vi "Function_Clamp #.vi"(8 "Error in":errorcluster, 9 "CoordSys In":T3 {"Measurement System"."Axis Reference" items=["Direct", "Indirect"]; "Measurement System"."Angle (deg)" format="%.2f"; "Measurement System"."Origin"."Y" format="%.2f"; "Measurement System"."Origin"."X" format="%.2f"; "Reference System"."Axis Reference" items=["Direct", "Indirect"]; "Reference System"."Angle (deg)" format="%.2f"; "Reference System"."Origin"."Y" format="%.2f"; "Reference System"."Origin"."X" format="%.2f"}, 10 "Data Cluster In":cluster{"Name":string, "Variant In":variant}, 11 "Image Src":T1) -> (0 "Error Out":errorcluster, 1 "Perpendicular Line(Offset)":T2, 2 "Fit Line(Offset)":T2, 3 "Result":cluster{"Name":string, "NG?":bool, "Score":dbl}, 4 "Time":u32)   [LabVIEW 2013]
uses:
  <vilib>/vision/Image Controls.llb/IMAQ Image.ctl
  Control/Control_Clamp.ctl
  <vilib>/vision/Measure.llb/Edge Options.ctl
  <vilib>/vision/Measure.llb/Edge Polarity.ctl
  <vilib>/vision/NI_Vision_Development_Module.lvlib
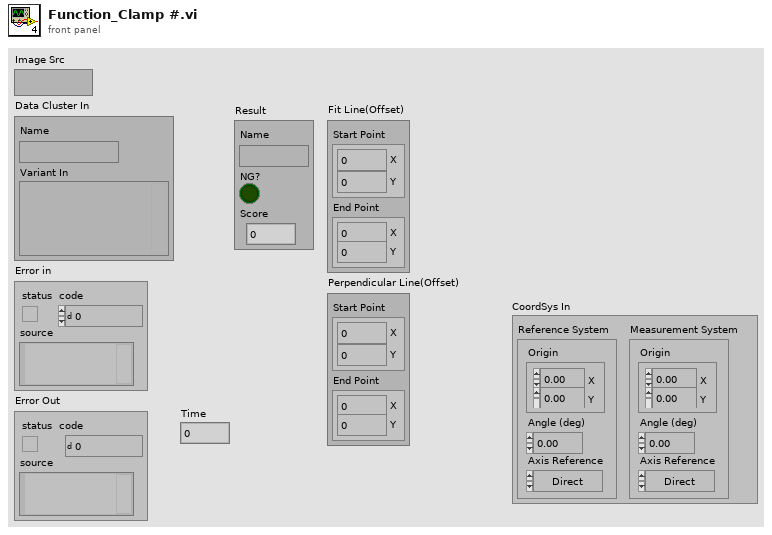
[diagram p1: front panel]
types:
  T1 = typedef "IMAQ Image.ctl" = refnum<image>
  T2 = cluster{"Start Point":cluster{"X":i32, "Y":i32}, "End Point":cluster{"X":i32, "Y":i32}}
  T3 = typedef "IMAQ Coordinate System" = cluster{"Reference System":cluster{"Origin":cluster{"X":sgl, "Y":sgl}, "Angle (deg)":sgl, "Axis Reference":u32}, "Measurement System":cluster{"Origin":cluster{"X":sgl, "Y":sgl}, "Angle (deg)":sgl, "Axis Reference":u32}}
  T4 = typedef "Control_Clamp.ctl" = cluster{"ROI Descriptor":cluster{"Global Rectangle":i32[], "Contours":cluster{"ID":enum32{"External", "Internal"}, "Type":u32, "Coordinates":i32[]}[]}, "Edge Options":cluster{"Edge Options":T5, "Scan Direction":u16, "Step Size":u32, "SD":dbl, "Auto":bool}, "條件(Clamp)":cluster{"間距":dbl}}
  T5 = typedef "Edge Options.ctl" = cluster{"Edge Polarity":T6, "Kernel Size":u32, "Width":u32, "Minimum Edge Strength":sgl, "Interpolation Type":enum32{"Zero Order", "Bilinear", "Quadratic", "Cubic", "Bilinear Fixed"}, "Data Processing Method":enum32{"Average", "Median"}}
  T6 = typedef "Edge Polarity.ctl" = u32
  T7 = cluster{"Global Rectangle":i32[], "Contours":cluster{"ID":enum32{"External", "Internal"}, "Type":u32, "Coordinates":i32[]}[]}
  T8 = cluster{"Origin":cluster{"X":sgl, "Y":sgl}, "Angle (deg)":sgl, "Axis Reference":u32}
  T9 = typedef "ROI Descriptor" = cluster{"Global Rectangle":i32[], "Contours":cluster{"ID":enum32{"External", "Internal"}, "Type":u32, "Coordinates":i32[]}[]}
  T10 = cluster{"Start Point":cluster{"X":sgl, "Y":sgl}, "End Point":cluster{"X":sgl, "Y":sgl}}
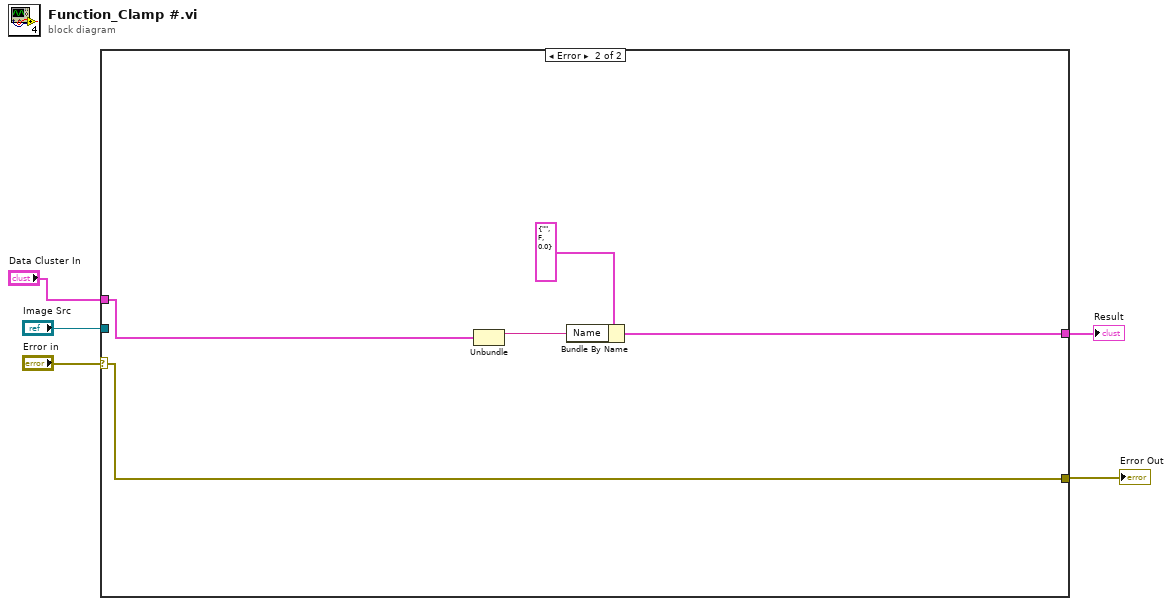
[diagram p0: block diagram]
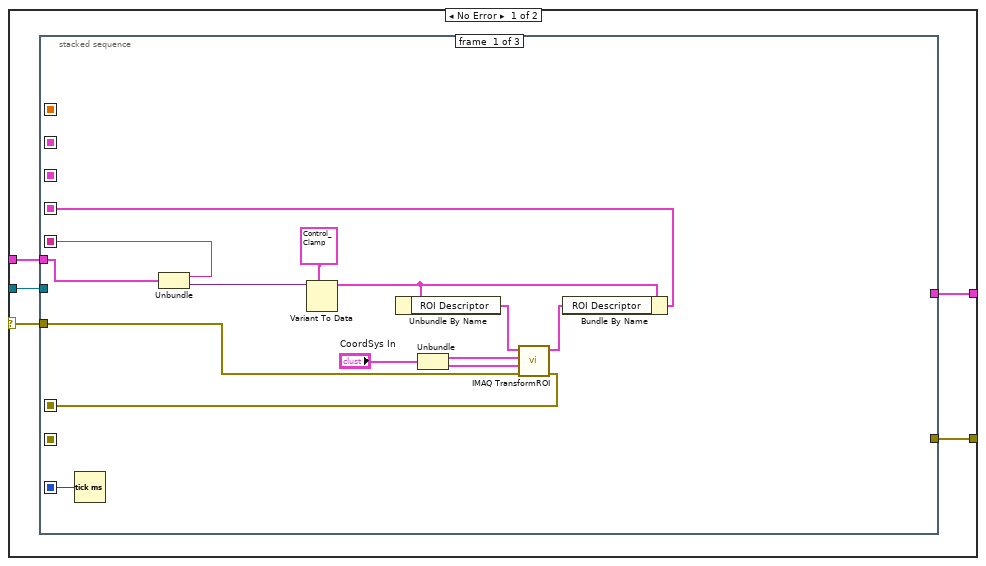
[diagram p2: hidden frame]
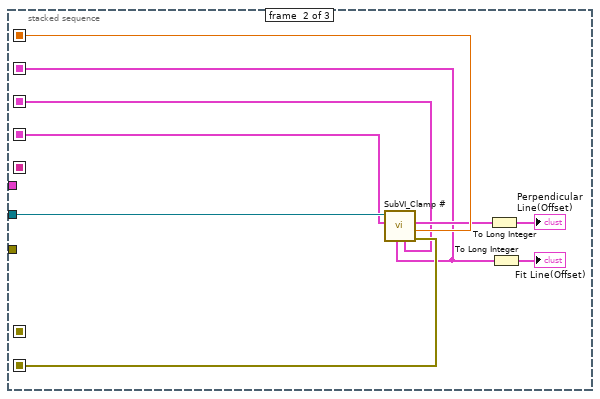
[diagram p3: hidden frame]
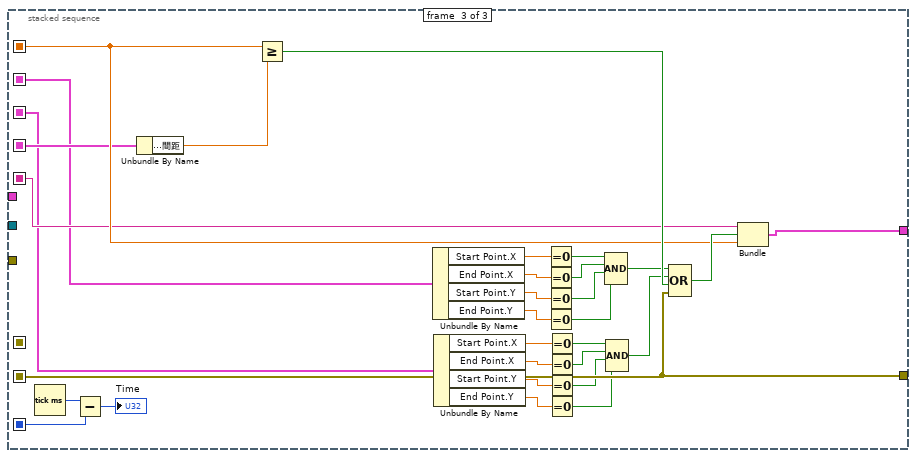
[diagram p4: hidden frame]
diagram:
  n1 = case shown="Error" "Error in" {
    selector: "Error in" -> [w8 w69]
    tunnel: "Image Src" -> [w10 _]
    tunnel: [w9 w69] -> w4
    tunnel: [w7 w66] -> w2
    tunnel: "Data Cluster In" -> [w6 w65]
    frame No Error {
      n2 = stacked-sequence {
        seq-local: [w16 _ _] -> [_ w31 w57]
        seq-local: [w23 _ _] -> [_ _ w63]
        seq-local: [_ w26 _] -> [_ _ w46]
        seq-local: [_ w32 _] -> [_ _ w58]
        seq-local: [_ w27 _] -> [_ _ w56]
        seq-local: [w21 _ _] -> [_ _ w55]
        seq-local: [w12 _ _] -> [_ _ _]
        seq-local: [_ w25 _] -> [_ _ w37]
        tunnel: w8 -> [w13 _ _]
        tunnel: w10 -> [_ w33 _]
        tunnel: [_ _ w56] -> w9
        tunnel: [_ _ w34] -> w7
        tunnel: w6 -> [w11 _ _]
        frame #0 {
          n3 = Tick Count (ms)() -> (millisecond timer value=w23:u32)
          n4 = Unbundle(w11) -> ("Name"=w21:string, "Variant In"=w24:variant)
          n5 = Variant To Data(type=T4 {"ROI Descriptor"={"Global Rectangle"=[], "Contours"=[]}, "Edge Options"={"Edge Options"={"Edge Polarity"=0, "Kernel Size"=0, "Width"=0, "Minimum Edge Strength"=0.0, "Interpolation Type"=enum."Zero Order", "Data Processing Method"=enum."Average"}, "Scan Direction"=0, "Step Size"=0, "SD"=0.0, "Auto"=FALSE}, "條件(Clamp)"={"間距"=0.0}} ("Parameter_Edge"), Variant=w24) -> (data=w15:T4)  [unwired: 1 in, 1 out]
          n6 = Unbundle By Name(w15) -> ("ROI Descriptor"=w17:T7)
          n7 = Unbundle("CoordSys In") -> ("Reference System"=w19:T8, "Measurement System"=w20:T8)
          n8 = call "IMAQ TransformROI"("error in (no error)"=w13, "New Reference"=w20, "Base Reference"=w19, "ROI Descriptor"=w17) -> ("error out"=w12:errorcluster, "ROI Descriptor out"=w14:T9)  [unwired: 6 in]
          n9 = Bundle By Name(cluster=w15, "ROI Descriptor"=w14) -> (w16:T4)
        }
        frame #1 {
          n10 = call "SubVI_Clamp #.vi"("Parameter_Edge"=w31, "Image in"=w33) -> ("error out"=w27:errorcluster, "Distance"=w32:dbl, "Perpendicular Line(Offset)"=w30:T10, "Fit Line 2"=w25:T10, "Fit Line"=w26:T10)  [unwired: 4 in, 1 out]
          n11 = To Long Integer(number=w30) -> (32bit integer=→"Perpendicular Line(Offset)":T2)
          n12 = To Long Integer(number=w26) -> (32bit integer=→"Fit Line(Offset)":T2)
        }
        frame #2 {
          n13 = Tick Count (ms)() -> (millisecond timer value=w64:u32)
          n14 = Subtract(x=w64, y=w63) -> (x-y=→"Time":u32)
          n15 = Unbundle By Name(w57) -> ("條件(Clamp).間距"=w59:dbl)
          n16 = Greater Or Equal?(x=w58, y=w59) -> (x >= y?=w60:bool)
          n17 = Unbundle By Name(w46) -> ("Start Point.X"=w47:sgl, "End Point.X"=w48:sgl, "Start Point.Y"=w49:sgl, "End Point.Y"=w50:sgl)
          n18 = Unbundle By Name(w37) -> ("Start Point.X"=w45:sgl, "End Point.X"=w44:sgl, "Start Point.Y"=w43:sgl, "End Point.Y"=w42:sgl)
          n19 = Equal To 0?(x=w47) -> (x = 0?=w51:bool)
          n20 = Equal To 0?(x=w48) -> (x = 0?=w52:bool)
          n21 = Equal To 0?(x=w49) -> (x = 0?=w53:bool)
          n22 = Equal To 0?(x=w50) -> (x = 0?=w54:bool)
          n23 = Equal To 0?(x=w45) -> (x = 0?=w41:bool)
          n24 = Equal To 0?(x=w44) -> (x = 0?=w40:bool)
          n25 = Equal To 0?(x=w43) -> (x = 0?=w39:bool)
          n26 = Equal To 0?(x=w42) -> (x = 0?=w38:bool)
          n27 = Compound Arithmetic op=AND(w51, w52, w53, w54) -> (w36:bool)
          n28 = Compound Arithmetic op=AND(w41, w40, w39, w38) -> (w35:bool)
          n29 = Compound Arithmetic op=OR(w36, w35, w60, w56) -> (w61:bool)
          n30 = Bundle("Name"=w55, w61, "Distance"=w58) -> (w34:cluster{"Name":string, bool, "Distance":dbl})  [unwired: 1 in]
        }
      }
    }
    frame Error {
      n31 = Unbundle(w65) -> ("Name"=w67:string)  [unwired: 1 out]
      n32 = Bundle By Name(cluster=cluster{"Name":string, bool, "Radius":dbl} {"Name"="", FALSE, "Radius"=0.0}, "Name"=w67) -> (w66:cluster{"Name":string, bool, "Radius":dbl})
    }
  }
  "Error Out" <- w4
  "Result" <- w2
